vi "New Assert Msg UT Setup.vi"(8 "error in (no error)":errorcluster) -> (0 "error out":errorcluster, 3 "Standard Display Configuration out":refnum<class "Standard Display Configuration.lvclass">)   [LabVIEW 2016]
uses:
  Core/Main Display/Display Configurations/Standard Display Configuration/Standard Display Configuration.lvclass
  Core/Assert API Components/Failure Actions.ctl
  Core/Assert API Components/Assert API Components.lvlib
  Core/Assert API Components/VI References.ctl
  Core/Assert API Components/Message Data.ctl
  C:/Users/ukhornp/Documents/Work/Projects/actor_assert_api/Core/Main Display/Display Configurations/Base Display Configuration.lvclass
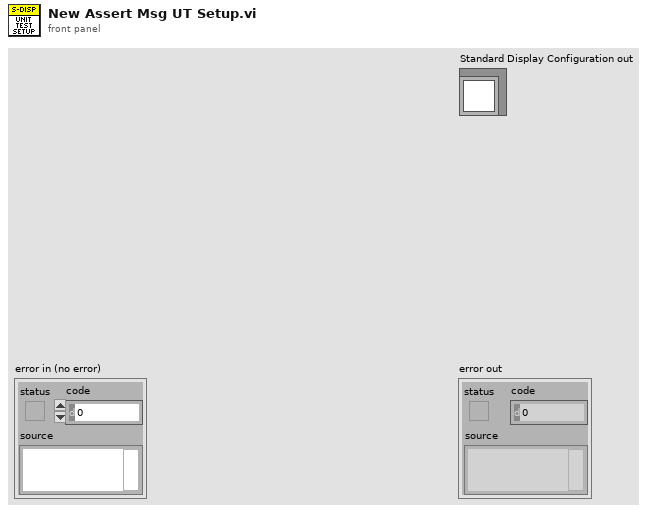
[diagram p1: front panel]
types:
  T1 = typedef "Assert API Components.lvlib/Message Data.ctl" = cluster{"Data Value":variant, "Last Update":timestamp, "Comment":string, "Evaluation String":string, "Status":bool, "Assert Name":string, "Failure Action":T2, "Assert VI Name":string, "Calling VI Name":string, "Assert VI UID":i32, "Top Level VI Name":string, "VI References":T3, "Assert Build Timestamp":timestamp, "Assert Builder User Name":string, "Data Type":string, "IP Address":string}
  T2 = typedef "Assert API Components.lvlib/Failure Actions.ctl" = enum16{"None", "Log To File", "Pause Execution", "Abort Execution"}
  T3 = typedef "Assert API Components.lvlib/VI References.ctl" = cluster{"Calling VI Ref":refnum<vi>, "Assert VI Ref":refnum<vi>}
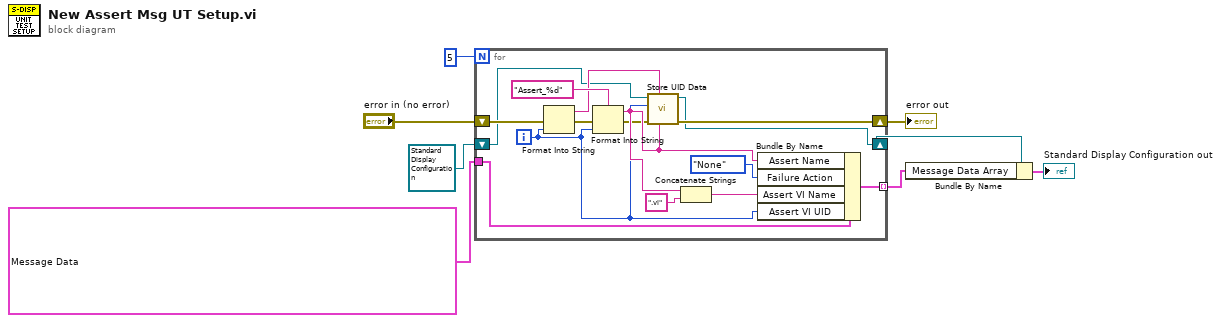
[diagram p0: block diagram]
diagram:
  n1 = for {
    N: 5 -> [_]
    tunnel: T1 {"Data Value"=variant, "Last Update"=timestamp(0 s since 1904-01-01), "Comment"="", "Evaluation String"="", "Status"=FALSE, "Assert Name"="", "Failure Action"=enum."None", "Assert VI Name"="", "Calling VI Name"="", "Assert VI UID"=0, "Top Level VI Name"="", "VI References"={"Calling VI Ref"=refnum, "Assert VI Ref"=refnum}, "Assert Build Timestamp"=timestamp(0 s since 1904-01-01), "Assert Builder User Name"="", "Data Type"="", "IP Address"=""} ("Assert Message") -> [w23]
    tunnel: [w18] -> w5 mode=indexing
    shift-right: [w10] -> w3
    shift-left: "error in (no error)" -> [w17]
    shift-right: [w9] -> w1
    shift-left: refnum<class "Standard Display Configuration.lvclass"> refnum ("Standard Display Configuration in") -> [w12]
    i -> [w13]
    n2 = Format Into String(error in=w17, w13) -> (resulting string=w14:string, error out=w16:errorcluster)  [unwired: 2 in]
    n3 = Format Into String(format string="Assert_%d", error in=w16, w13) -> (resulting string=w15:string, error out=w11:errorcluster)  [unwired: 1 in]
    n4 = call "Store UID Data.vi"("Assert Name"=w15, "UID Value"=w14, "error in (no error)"=w11, "Assert Count Value"=w13, "Standard Display Configuration in"=w12) -> ("error out"=w10:errorcluster, "Standard Display Configuration out"=w9:refnum<class "Standard Display Configuration.lvclass">)  [unwired: 5 in]
    n5 = Concatenate Strings(w15, ".vi" ("string")) -> (w19:string)
    n6 = Bundle By Name(cluster=w23, "Assert Name"=w15, "Failure Action"=Failure_Actions."None", "Assert VI Name"=w19, "Assert VI UID"=w13) -> (w18:T1)
  }
  "error out" <- w3
  n7 = Bundle By Name(cluster=w1, "Message Data Array"=w5) -> (→"Standard Display Configuration out":cluster{})
